vi "Build LT Evaluation String.vi"(8 "error in (no error)":errorcluster, 11 "Test in":refnum<class "Test.lvclass">) -> (0 "error out":errorcluster, 2 "Equals Evaluation String":string)   [LabVIEW 2018, in "Test.lvclass"]
doc: "Builds an evaluation string for a Greater Than test - can be used across different data type child classes within the test class structure."
uses:
  Test.lvclass
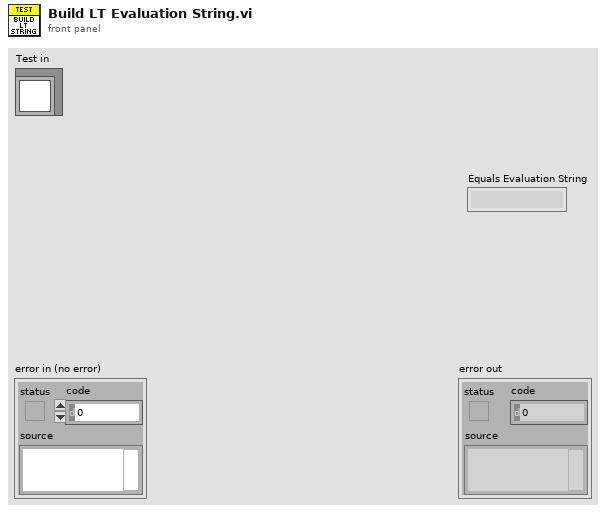
[diagram p1: front panel]
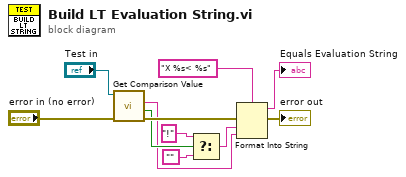
[diagram p0: block diagram]
diagram:
  n1 = call "Get Comparison Value.vi"("error in (no error)"="error in (no error)", "Test in"="Test in") -> ("error out"=w7:errorcluster, "Invert Result"=w6:bool, "Data String"=w5:string)  [unwired: 7 in]
  n2 = Select(t="!", s=w6, f="") -> (s? t:f=w8:string)
  n3 = Format Into String(format string="X %s< %s", error in=w7, w8, w5) -> (resulting string=→"Equals Evaluation String":string, error out=→"error out":errorcluster)  [unwired: 1 in]
